vi "addNewElement.vi"(6 "firstItem? (F)":bool, 8 "error in (no error)":errorcluster, 9 "prevObjRef":refnum<vi>, 10 "clusterInfo.reference":refnum<vi>, 11 "Element in":refnum<class "Element.lvclass">) -> (0 "error out":errorcluster, 3 "Element out":refnum<class "Element.lvclass">)   [LabVIEW 2012, in "Element.lvclass"]
uses:
  Element.lvclass
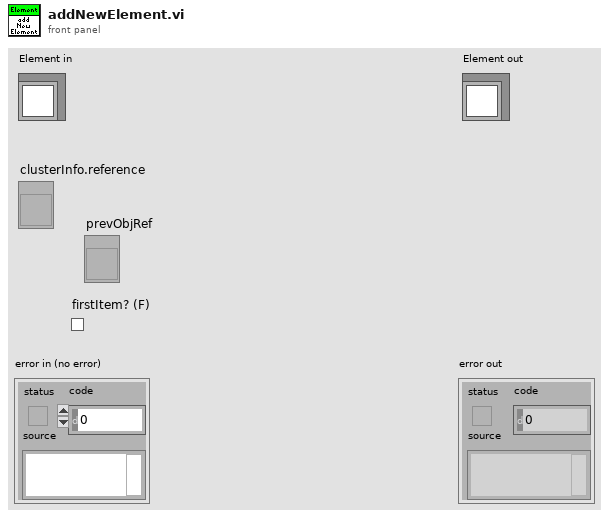
[diagram p1: front panel]
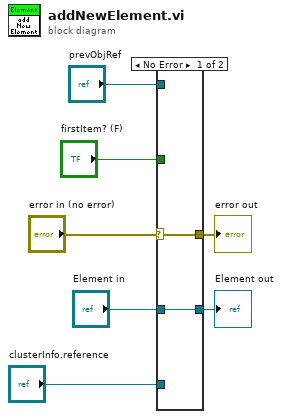
[diagram p0: block diagram]
diagram:
  n1 = case shown="No Error" "error in (no error)" {
    selector: "error in (no error)" -> [w8 w11]
    tunnel: [w8 w11] -> w6
    tunnel: [w9 w10] -> w4
    tunnel: "Element in" -> [w9 w10]
    tunnel: "clusterInfo.reference" -> [_ _]
    tunnel: "firstItem? (F)" -> [_ _]
    tunnel: "prevObjRef" -> [_ _]
    frame No Error {
    }
    frame Error {
    }
  }
  "error out" <- w6
  "Element out" <- w4
